vi "Set Message Text.vi"(8 "error in (no error)":errorcluster, 9 "Message":string, 10 "Subject":string, 11 "Mail in":refnum<class "Mail.lvclass">) -> (0 "error out":errorcluster, 3 "Mail out":refnum<class "Mail.lvclass">)   [LabVIEW 2023, in "HardwareAbstractionLayer_LVOOP.lvlib" / "Mail.lvclass"]
uses:
  Mail.lvclass
  Mail.lvclass/Mail.ctl
  <vilib>/smtpClient/LabVIEWSMTPClient.lvlib
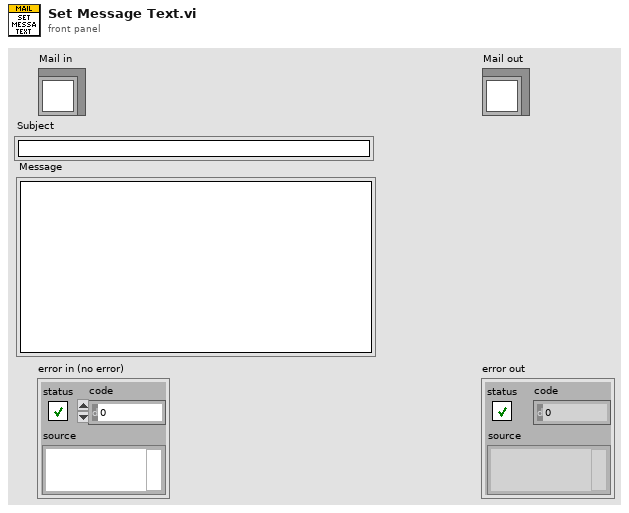
[diagram p1: front panel]
types:
  T1 = typedef "LabVIEWSMTPClient.lvlib/SmtpClientHandle.ctl" = refnum<k1>
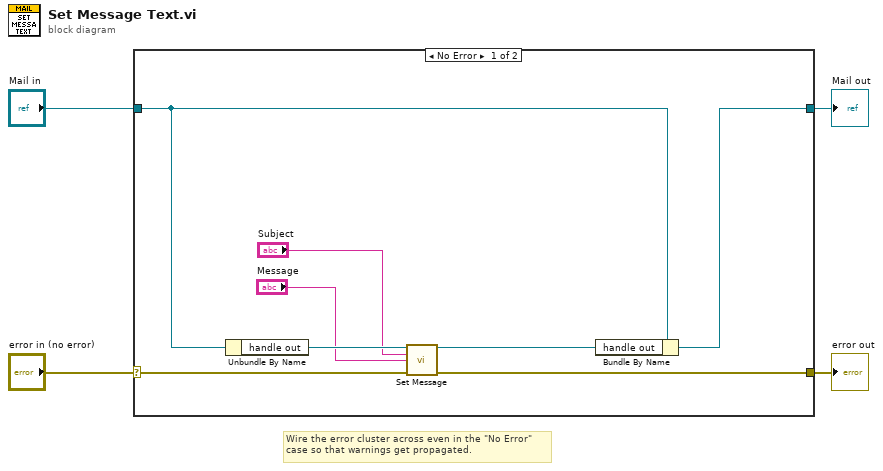
[diagram p0: block diagram]
diagram:
  # "Wire the error cluster across even in the \"No Error\"\ncase so that warnings get propagated."
  n1 = case shown="No Error" "error in (no error)" {
    selector: "error in (no error)" -> [w12 w14]
    tunnel: [w11 w14] -> w3
    tunnel: [w7 w13] -> w1
    tunnel: "Mail in" -> [w8 w13]
    frame No Error {
      n2 = Unbundle By Name(w8) -> ("handle out"=w10:T1)
      n3 = call-poly <vilib>:"Set Message.vi"("handle in"=w10, "subject"="Subject", "plain text message"="Message", "error in (no error)"=w12) -> ("handle out"=w9:T1, "error out"=w11:errorcluster)  [unwired: 10 in]
      n4 = Bundle By Name(cluster=w8, "handle out"=w9) -> (w7:refnum<class "Mail.lvclass">)
    }
    frame Error {
    }
  }
  "error out" <- w3
  "Mail out" <- w1
